vi "Get Gear Ratios.vi"(8 "error in (no error)":errorcluster, 11 "Finger in":refnum<class "Finger.lvclass">) -> (0 "error out":errorcluster, 2 "gear ratios":dbl[](array[numeric]), 3 "Finger out":refnum<class "Finger.lvclass">)   [LabVIEW 2011, in "Finger.lvclass"]
uses:
  Finger.lvclass
  Finger.lvclass/Finger.ctl
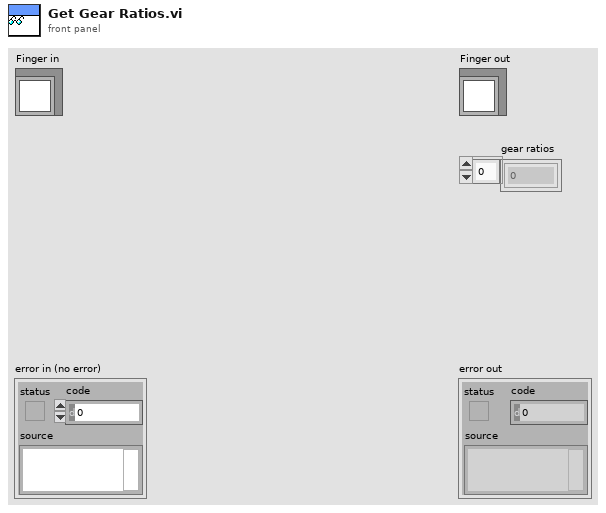
[diagram p1: front panel]
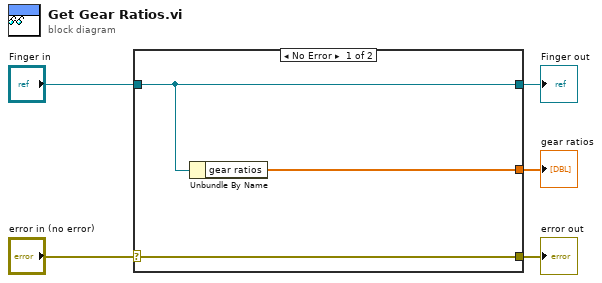
[diagram p0: block diagram]
diagram:
  n1 = case shown="No Error" "error in (no error)" {
    selector: "error in (no error)" -> [w8 w9]
    tunnel: [w8 w9] -> w4
    tunnel: [w7 w10] -> w2
    tunnel: "Finger in" -> [w7 w10]
    tunnel: [w6 _] -> w1
    frame No Error {
      n2 = Unbundle By Name(w7) -> ("gear ratios"=w6:dbl[])
    }
    frame Error {
    }
  }
  "error out" <- w4
  "Finger out" <- w2
  "gear ratios" <- w1
